vi "Write Efuse Multiplier.vi"(10 "Efuse Multiplier":T1, 11 "Toggle 6 in":refnum<class "Toggle 6.lvclass">) -> (3 "Toggle 6 out":refnum<class "Toggle 6.lvclass">)   [LabVIEW 2020, in "Toggle 6.lvclass"]
uses:
  Toggle 6.lvclass
  Controls/EFuse modes enum.ctl
  Toggle 6.lvclass/Toggle 6.ctl
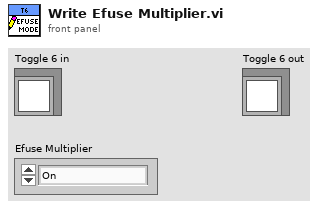
[diagram p1: front panel]
types:
  T1 = typedef "Toggle 6.lvclass/EFuse modes enum.ctl" = enum16{"On", "Off", "Both On and Off"}
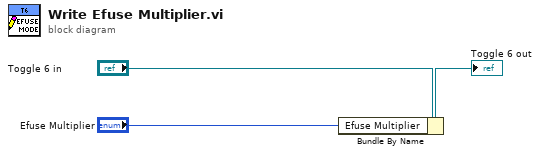
[diagram p0: block diagram]
diagram:
  n1 = Bundle By Name(cluster="Toggle 6 in", "Efuse Multiplier"="Efuse Multiplier") -> (→"Toggle 6 out":refnum<class "Toggle 6.lvclass">)
